vi "FRCts20_Backend_GetTeamList.vi"(8 "error in (no error)":errorcluster, 9 "Key":string, 11 "Competitions":T1) -> (0 "error out":errorcluster)   [LabVIEW 2014, in "FRCts20_Backend_Engine_Deprecated.lvlib"]
uses:
  FRCts20_Backend_Engine_Deprecated.lvlib
  FRCts20_Backend_Engine.lvlib
  FRCts20_Backend_FGVOperation.ctl
  FRCts20_Backend_Competition_Info.ctl
  FRCts20_Backend_Controls.lvlib
  FRCts20_Backend_Division_Info.ctl
  FRCts20_Backend_Team_Info.ctl
  FRCts20_Backend_Note.ctl
  FRCts20_Backend_Note_list.ctl
  FRCts20_Backend_request_info.ctl
  FRCts20_Backend_IssueDfn.ctl
  FRCts20_Backend_IssueTeamList.ctl
  FRCts20_Backend_TeamDfn.ctl
  FRCts20_Backend_TeamDataDfn.ctl
  FRCts20_Backend_Division.ctl
  FRCts20_Backend_Division_List.ctl
  FRCts20_Backend_Competition.ctl
  FRCts20_Backend_Competition_List.ctl
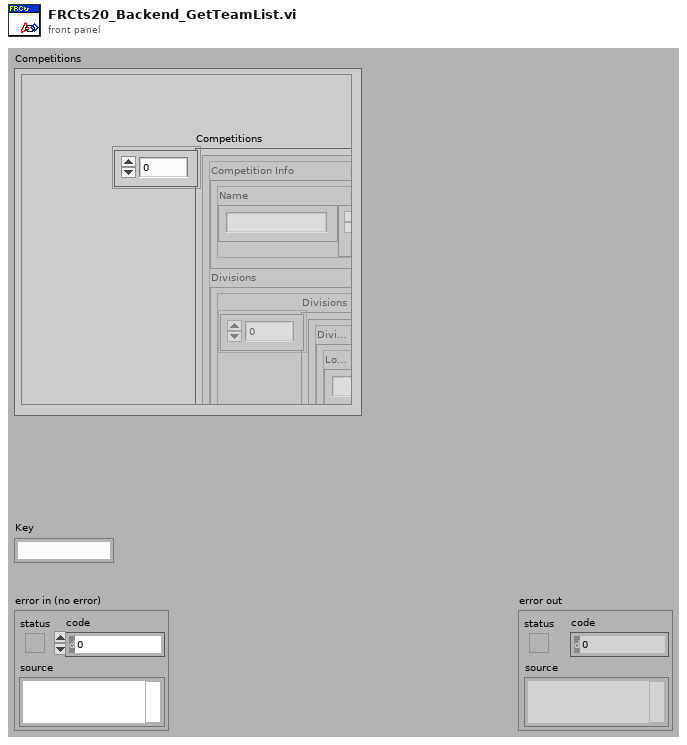
[diagram p1: front panel]
types:
  T1 = typedef "FRCts20_Backend_Controls.lvlib/FRCts20_Backend_Competition_List.ctl" = cluster{"Competitions":T2[]}
  T2 = typedef "FRCts20_Backend_Controls.lvlib/FRCts20_Backend_Competition.ctl" = cluster{"Competition Info":T3, "Divisions":T4}
  T3 = typedef "FRCts20_Backend_Controls.lvlib/FRCts20_Backend_Competition_Info.ctl" = cluster{"Name":string, "Start Date":timestamp, "Duration":u8}
  T4 = typedef "FRCts20_Backend_Controls.lvlib/FRCts20_Backend_Division_List.ctl" = cluster{"Divisions":T5[]}
  T5 = typedef "FRCts20_Backend_Controls.lvlib/FRCts20_Backend_Division.ctl" = cluster{"Division Info":T6, "TeamData":T7}
  T6 = typedef "FRCts20_Backend_Controls.lvlib/FRCts20_Backend_Division_Info.ctl" = cluster{"Location":string}
  T7 = typedef "FRCts20_Backend_Controls.lvlib/FRCts20_Backend_TeamDataDfn.ctl" = cluster{"Team":T8[]}
  T8 = typedef "FRCts20_Backend_Controls.lvlib/FRCts20_Backend_TeamDfn.ctl" = cluster{"Team Info":T9, "IssueList":T10}
  T9 = typedef "FRCts20_Backend_Controls.lvlib/FRCts20_Backend_Team_Info.ctl" = cluster{"TeamNumber":u16, "SWType":string}
  T10 = typedef "FRCts20_Backend_Controls.lvlib/FRCts20_Backend_IssueTeamList.ctl" = cluster{"Issues":T11[]}
  T11 = typedef "FRCts20_Backend_Controls.lvlib/FRCts20_Backend_IssueDfn.ctl" = cluster{"Notes":T12, "Info":T14}
  T12 = typedef "FRCts20_Backend_Controls.lvlib/FRCts20_Backend_Note_list.ctl" = cluster{"Notes":T13[]}
  T13 = typedef "FRCts20_Backend_Controls.lvlib/FRCts20_Backend_Note.ctl" = cluster{"Time Entered":timestamp, "Author":string, "Text":string}
  T14 = typedef "FRCts20_Backend_Controls.lvlib/FRCts20_Backend_request_info.ctl" = cluster{"Status":enum16{"Open", "In Work", "Closed"}, "Open Date":timestamp, "Description":string, "Last Update":timestamp, "Closed Date":timestamp, "Solution Index":i32}
  T15 = typedef "FRCts20_Backend_Engine.lvlib/FRCts20_Backend_FGVOperation.ctl" = enum16{"Initialize", "EnqueueMessage", "EnqueueDataReturn", "FlushMessage", "FlushDataReturn"}
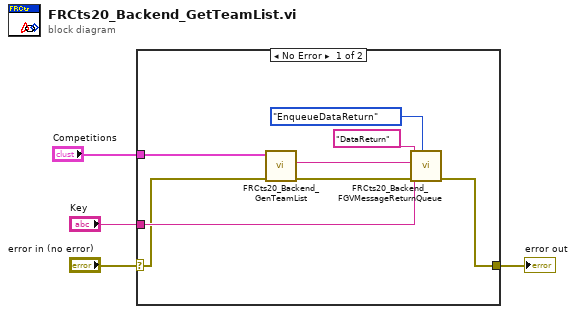
[diagram p0: block diagram]
diagram:
  n1 = case shown="No Error" "error in (no error)" {
    selector: "error in (no error)" -> [w8 w13]
    tunnel: [w9 w13] -> w3
    tunnel: "Key" -> [w10 _]
    tunnel: "Competitions" -> [w5 _]
    frame No Error {
      n2 = call "FRCts20_Backend_GenTeamList.vi"("error in (no error)"=w8, "Competitions"=w5) -> ("error out"=w7:errorcluster, "TeamList_Flattened"=w6:string)  [unwired: 7 in, 1 out]
      n3 = call "FRCts20_Backend_FGVMessageReturnQueue.vi"("Operation"=FRCts20_Backend_FGVOperation."EnqueueDataReturn", "error in (no error)"=w7, "Key"=w10, "Message Value"=w6, "Message Name"="DataReturn") -> ("error out"=w9:errorcluster)  [unwired: 3 in, 1 out]
    }
    frame Error {
    }
  }
  "error out" <- w3
